vi "Barcode scan.vi"(10 "Scan Data":refnum<vi>) -> ()   [LabVIEW 2015]
uses:
  <vilib>/Instr/_visa.llb/VISA Configure Serial Port (Instr).vi
  Galobal variable_TI.vi
panel:
  out "read buffer":string
  out "error out 4":errorcluster
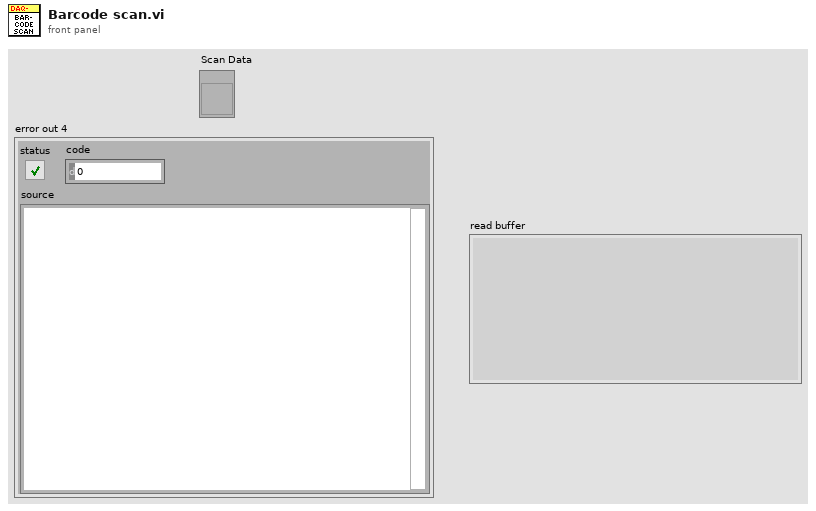
[diagram p1: front panel]
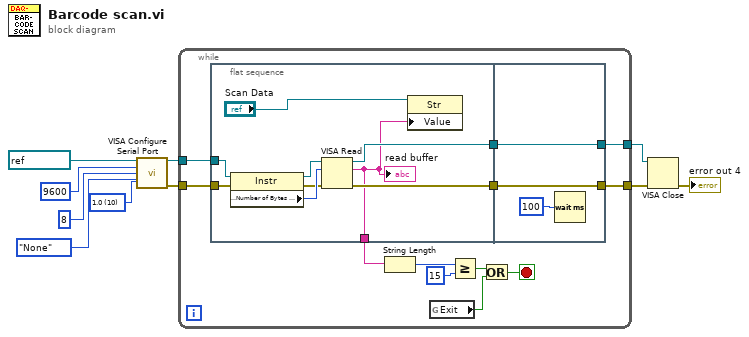
[diagram p0: block diagram]
diagram:
  w1 = u16 10 items=["1.0"=10, "1.5"=15, "2.0"=20] ("stop bits (10: 1 bit)")
  n1 = call-poly "VISA Configure Serial Port"("VISA resource name"=refnum<visa-resource-name> "COM4", "baud rate (9600)"=u32 9600, "data bits (8)"=u16 8, "parity (0:none)"=enum16{"None", "Odd", "Even", "Mark", "Space"}."None", "stop bits (10: 1 bit)"=w1) -> ("VISA resource name out"=w9:refnum<visa-resource-name>, "error out"=w8:errorcluster)  [unwired: 4 in, 5 out]
  n2 = while {
    tunnel: w9 -> [w20]
    tunnel: [w18] -> w6
    tunnel: w8 -> [w19]
    tunnel: [w17] -> w5
    stop <- w12 stop-if-true
    n3 = flat-sequence {
      tunnel: w20 -> [w28]
      tunnel: w19 -> [w26]
      tunnel: [w31] -> w22
      tunnel: [w30] -> w21
      tunnel: [w23] -> w16
      tunnel: w22 -> [w34]
      tunnel: [w34] -> w18
      tunnel: w21 -> [w33]
      tunnel: [w33] -> w17
      frame #0 {
        n4 = property class="Instr"(reference=w28, error in=w26) -> (reference out=w27:refnum<visa-resource-name>, error out=w25:errorcluster, "Serial Settings:Number of Bytes at Serial Port"=w29:u32)
        n5 = VISA Read(VISA resource name=w27, byte count=w29, error in (no error)=w25) -> (VISA resource name out=w31:refnum<visa-resource-name>, read buffer=w23:string, error out=w30:errorcluster)  [unwired: 1 out]
        "read buffer" <- w23
        n6 = property class="Str"(reference="Scan Data", "Value"=w23) -> ()  [unwired: 1 in, 2 out]
      }
      frame #1 {
        n7 = Wait (ms)(milliseconds to wait=u32 100) -> ()  [unwired: 1 out]
      }
    }
    n8 = String Length(string=w16) -> (length=w15:i32)
    n9 = global read "Galobal variable_TI.vi" "Exit"() -> (w11:bool)
    n10 = Greater Or Equal?(x=w15, y=15) -> (x >= y?=w13:bool)
    n11 = Or(x=w13, y=w11) -> (x .or. y?=w12:bool)
  }
  n12 = VISA Close(VISA resource name=w6, error in (no error)=w5) -> (error out=→"error out 4":errorcluster)
